vi "写入地址.vi"(8 "error in (no error)":errorcluster caption="错误输入（无错误）", 10 "地址":string="localhost", 11 "LS-H600-TCP Client输入":refnum<class "LS-H600-TCP Client.lvclass">) -> (0 "error out":errorcluster caption="错误输出", 3 "LS-H600-TCP Client输出":refnum<class "LS-H600-TCP Client.lvclass">)   [LabVIEW 2022 SP3, in "LS-H600-TCP Client.lvlib" / "LS-H600-TCP Client.lvclass"]
uses:
  LS-H600-TCP Client.lvclass
  LS-H600-TCP Client.lvclass/LS-H600-TCP Client.ctl
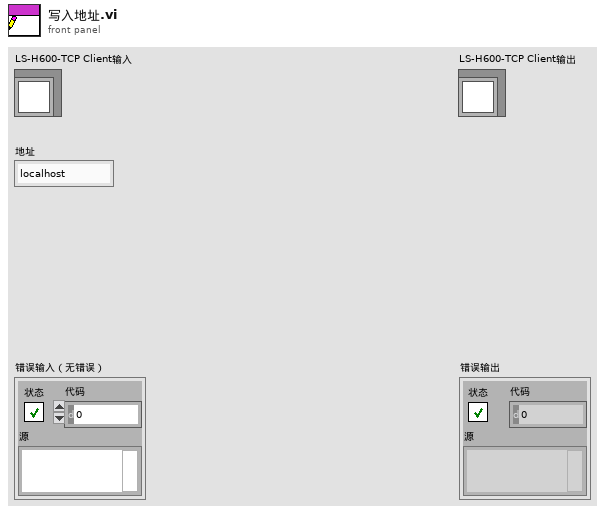
[diagram p1: front panel]
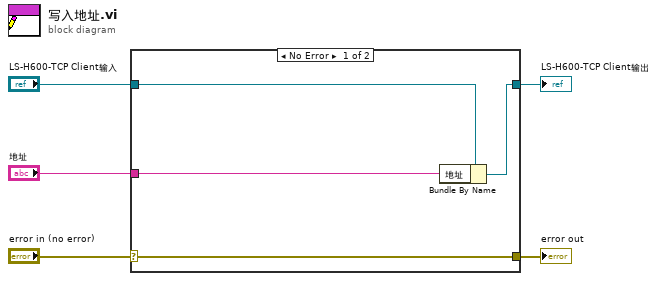
[diagram p0: block diagram]
diagram:
  n1 = case shown="No Error" "error in (no error)" {
    selector: "error in (no error)" -> [w9 w10]
    tunnel: [w9 w10] -> w4
    tunnel: [w7 w11] -> w2
    tunnel: "LS-H600-TCP Client输入" -> [w8 w11]
    tunnel: "地址" -> [w6 _]
    frame No Error {
      n2 = Bundle By Name(cluster=w8, "地址"=w6) -> (w7:refnum<class "LS-H600-TCP Client.lvclass">)
    }
    frame Error {
    }
  }
  "error out" <- w4
  "LS-H600-TCP Client输出" <- w2
